vi "GPS - Initialise_SubVI.vi"(8 "error in (no error)":errorcluster) -> (0 "error out":errorcluster, 3 "VISA Refnum out":refnum<visa-resource-name>)   [LabVIEW 2021]
uses:
  <vilib>/Instr/_visa.llb/VISA Configure Serial Port (Instr).vi
  <vilib>/myRIO/Instrument Drivers/Onboard IO/UART/typedef/VISA Configuration.ctl
  <vilib>/myRIO/Instrument Drivers/Onboard IO/UART/UART.lvlib
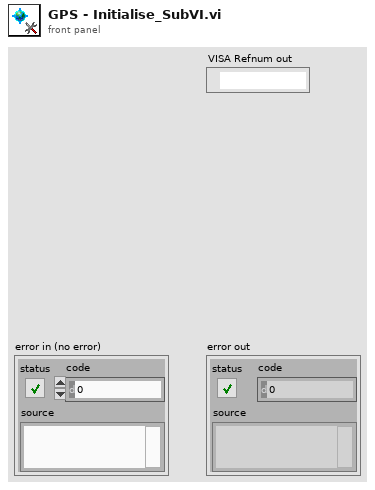
[diagram p1: front panel]
types:
  T1 = typedef "UART.lvlib/VISA Configuration.ctl" = cluster{"baud rate (9600)":u32, "data bits (8)":u16, "parity (0:none)":enum16{"None", "Odd", "Even", "Mark", "Space"}, "stop bits (10: 1 bit)":u16, "flow control (0:none)":u16, "termination char\n(0xA = '\\n' = LF) ":u8, "Enable Termination\nChar (T)":bool, "timeout (10sec)":u32}
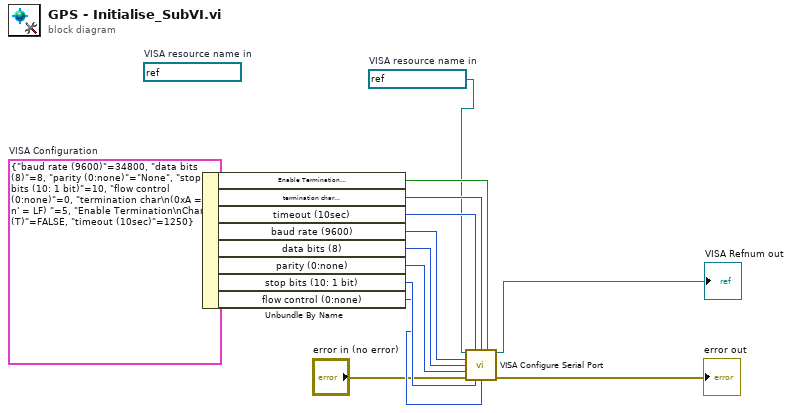
[diagram p0: block diagram]
diagram:
  w2 = refnum<visa-resource-name> "ASRL1::INSTR"  # VISA resource name in
  (unwired) refnum<visa-resource-name> "ASRL2::INSTR"  # VISA resource name in
  w3 = T1 {"baud rate (9600)"=34800, "data bits (8)"=8, "parity (0:none)"=enum."None", "stop bits (10: 1 bit)"=10, "flow control (0:none)"=0, "termination char\n(0xA = '\\n' = LF) "=5, "Enable Termination\nChar (T)"=FALSE, "timeout (10sec)"=1250}  # VISA Configuration
  n1 = Unbundle By Name(w3) -> ("Enable Termination\nChar (T)"=w5:bool, "termination char\n(0xA = '\\n' = LF)"=w6:u8, "timeout (10sec)"=w7:u32, "baud rate (9600)"=w12:u32, "data bits (8)"=w11:u16, "parity (0:none)"=w10:enum16{"None", "Odd", "Even", "Mark", "Space"}, "stop bits (10: 1 bit)"=w9:u16, "flow control (0:none)"=w8:u16)
  n2 = call-poly "VISA Configure Serial Port"("VISA resource name"=w2, "timeout (10sec)"=w7, "termination char\n(0xA = '\\n' = LF)"=w6, "Enable Termination\nChar (T)"=w5, "baud rate (9600)"=w12, "data bits (8)"=w11, "parity (0:none)"=w10, "error in (no error)"="error in (no error)", "stop bits (10: 1 bit)"=w9, "flow control (0:none)"=w8) -> ("VISA resource name out"=→"VISA Refnum out":refnum<visa-resource-name>, "error out"=→"error out":errorcluster)  [unwired: 4 in]
